vi "Transfer_Curve_2_2400.vi"(0 "File Path":path=path "C:/DATA/raj/transferdump.txt.txt", 1 "V_G Start":dbl=-0.7 format="%#.3g", 3 "V_G Finish":dbl=0.4 format="%#.3g", 4 "V_G Step Size":dbl=0.05 format="%#.3g", 5 "Preread delay (ms)":dbl=10000.0 format="%.2f", 7 "Delay between \naverages (ms)":dbl=200.0 format="%#.3f", 8 "Keithley 237 GPIB address":string="17", 9 "Software Averages":i16=5, 12 "2400":refnum<visa-resource-name>="GPIB0::24::INSTR", 13 "First bias settle (ms)":dbl=60000.0 format="%#.2f", 15 "Current Compliance\nLimit (A) Ke2400":dbl=0.1 format="%#.3e", 18 "Dimensions":T1(ring), 24 "Voltage Compliance Limit 237 (V)":dbl=10.0 format="%#.3f", 25 "Current Compliance\nLimit 237 (A)":dbl=0.1 format="%#.3f", 27 "V_DS":dbl=-0.6 format="%#_13g") -> ()   [LabVIEW 2018]
uses:
  <vilib>/Utility/file.llb/Write Delimited Spreadsheet (string).vi
  Instance           1 16Saved   JV curve .vi
  <instrlib>/Keithley 24XX/Public/Data/Read (Single Point).vi
  <vilib>/Analysis/NI_AALBase.lvlib
  <instrlib>/Keithley 24XX/Keithley 24XX.lvlib
panel:
  in  "2401":refnum<visa-resource-name>="GPIB0::22::INSTR"
  in  "Quick Burn In?":bool
  out "timer":dbl format="%#_6f"
  out "Keithley 2400":cluster{dbl[], dbl[]}(graph)={[-2.0, -1.9, -1.8, -1.7, -1.6, -1.5], [-6.6965744e-11, -6.7804984e-11, -6.685451799999999e-11, -6.6450076e-11, -6.5125542e-11, -6.7339852e-11]}
  out "I_G (A)":dbl=-6.642986e-11 format="%.2e"
  in  "Autozero?":u16(ring) items=["On", "Off", "Once"]
  in  "Measurement Speed (1 PLC)":dbl=1.0 format="%.2g"
  in  "Manual Range (Max I)":dbl=1.0
  in  "Enable Meas Auto Range":bool=TRUE
  in  "Source Mode":u16(ring) items=["Voltage", "Current"]
  in  "Return Sweep?":bool=TRUE
  out "I_DS":dbl=-1.38e-12 format="%.2e"
  out "Outputfile":path=path "C:/DATA/Mark Ziffer/test10"
  in  "Abort Scan":bool=TRUE
  out "V_G":dbl=-1.5 format="%#.2f"
  out "Keithley 237":cluster{dbl[], dbl[]}(graph)={[-2.0, -1.9, -1.8, -1.7, -1.6, -1.5], [-6.720000000000001e-13, -2.18e-13, -2.7599999999999993e-13, -8.999999999999998e-14, -1.3999999999999998e-13, -1.3800000000000002e-13]}
  # "Transfer Curve\nbased on  EL_photocurrent_JV.vi for controlling 2 Ketthleys\n\n9/2017 MZ"
  # "Software Settings"
  # "Ke237 Settings"
  # "Ke2400 Settings"
  # "Notes for IV Scan\n\n2010.07.06 - add absolute value plotter to look at log-scale current\n2010.01.07 - Modified file headers for distinguihing when imported to Igor Pro - the prefix of each header will be the file name.\n2009.01.15 - I updated the code to run on the VISA driver convention. I also modified the file saving and the option to set the\n                      graph display.\n2008.12.01 - I fixed an issue with calculations of J. It was mis-wired to divide current by wavelength, rather than active area.  BM\n\n=========================\nI added the functionality to calculate the fill factor, rectification ratio, short circuit current density, and open circuit voltage. \nAdditionally, current density (mA/cm^2) is reported in the plot window and column B of the data file, and the current (A) has been \nmoved to column C. Open circuit voltage is linearly interpolated. The max power point (mpp) for calculating fill factor is taken as \nthe data point with the highest I-V product, so this makes it only as accurate as your voltage step size, but should be fine for a decent \ndevice on the 50 mV default step size.\n\nIf you know how to use the previous versions of IV scan, \nmake sure you set these parameters before you scan:\n1) Recftification Ratio Bias - this is the +/- bias value you wish to record a rectification ratio at.\n2) Effective Area - this is the area in cm^2 of the diode mask (photoactive area) when measuring under illumination or the measured \n     area of the electrode overlap when measured in dark (regular active area).\n3) Do you want to record a separate data file for the calculated characteristics? If so, make sure the switch is on.\n\nAs of today, I couldn't figure out how to append the computed characteristics to the I-V file without experiencing formating issues, so\nI opted to just create a separate file if you want to save that info. Feel free to fix this if you know how. Check tab 3 > tab 2 > tab 9 in the\nblock diagram.\n\n2008-04-15\nB MacLeod"
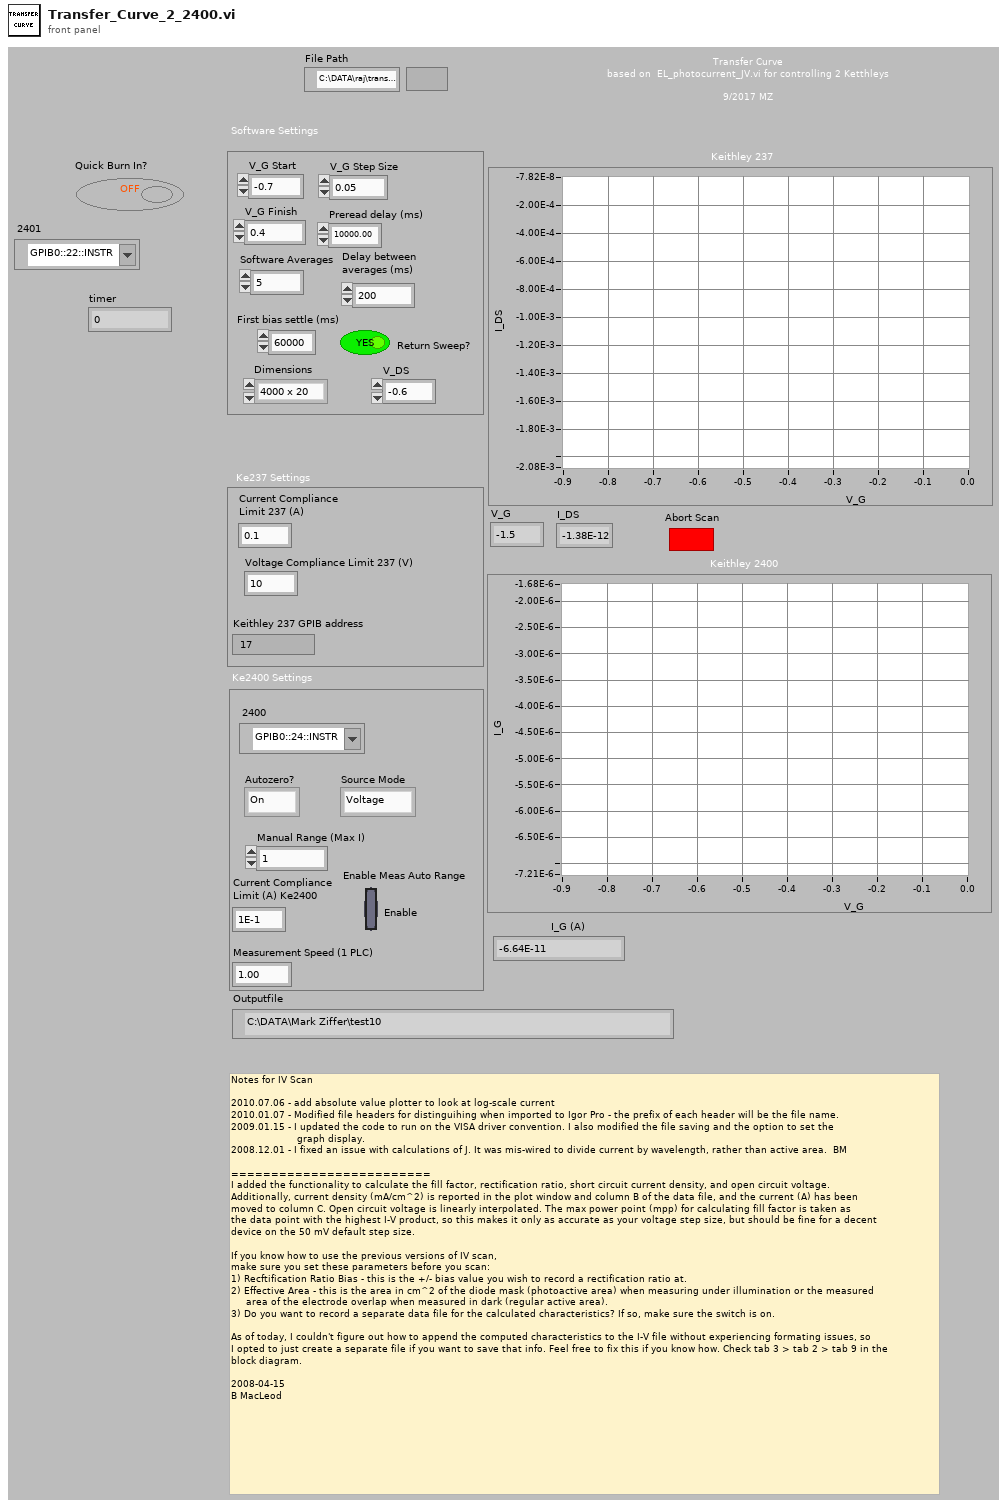
[diagram p1: front panel]
types:
  T1 = enum16{"4000 x 20", "2000 x 20", "1000 x 20", "800 x 20", "400 x 20", "200 x 20", "100 x 20"}
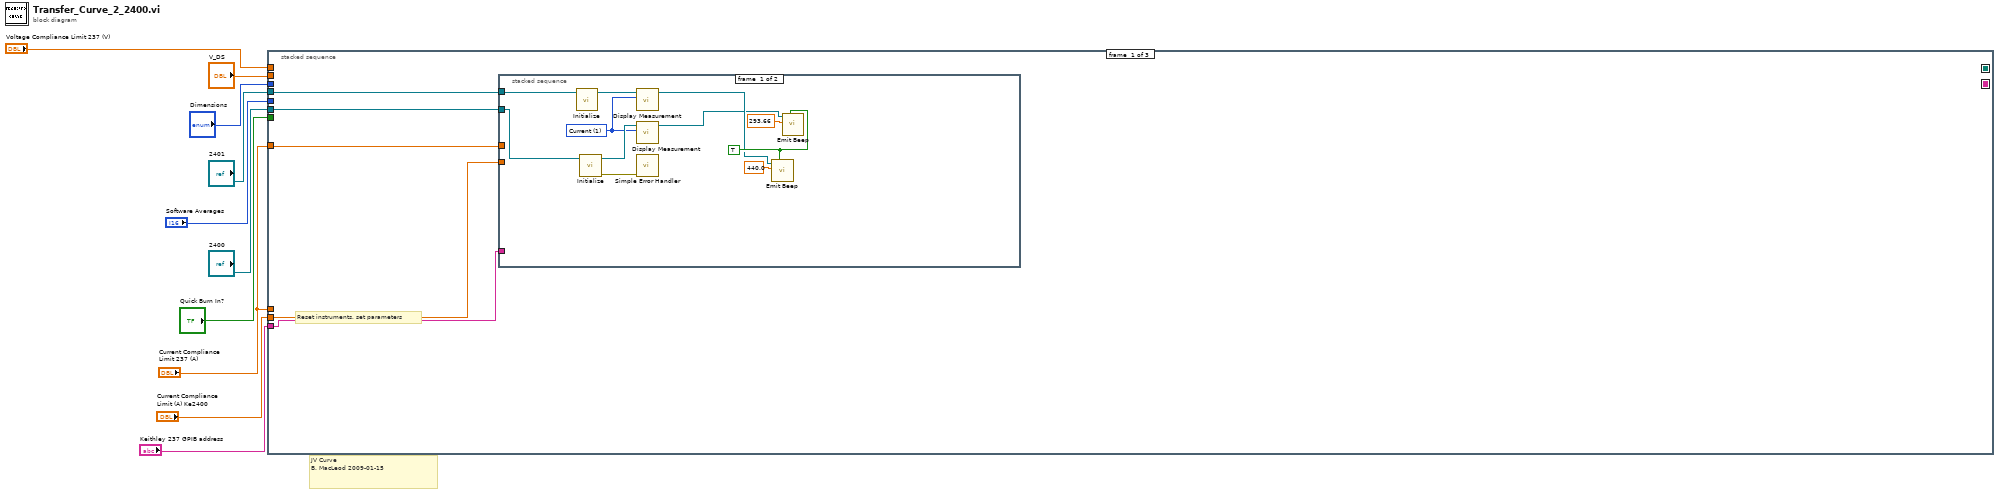
[diagram p0: block diagram]
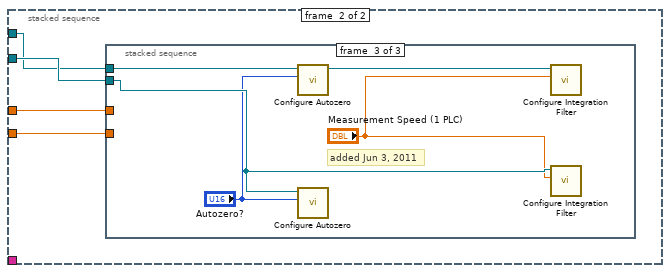
[diagram p2: hidden frame]
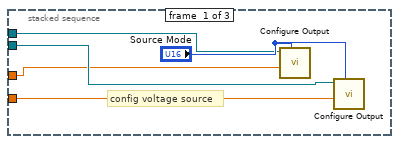
[diagram p3: hidden frame]
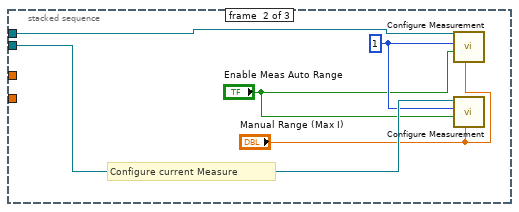
[diagram p4: hidden frame]
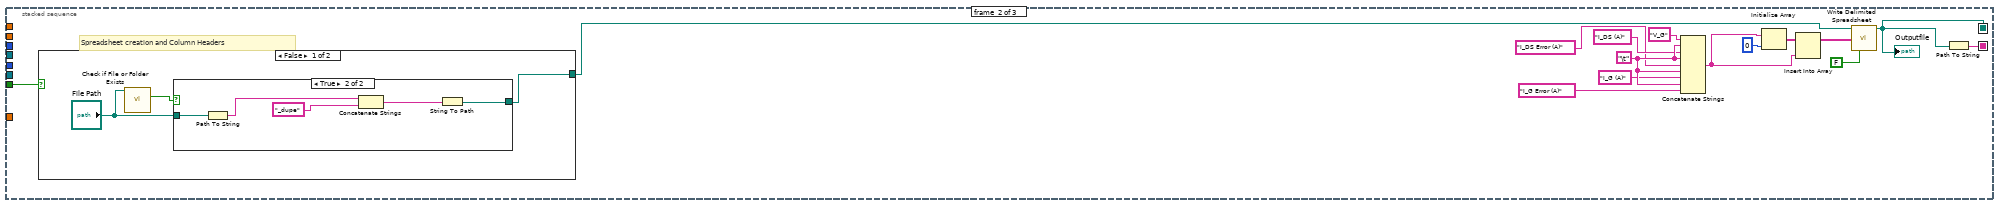
[diagram p5: hidden frame]
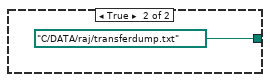
[diagram p7: hidden frame]
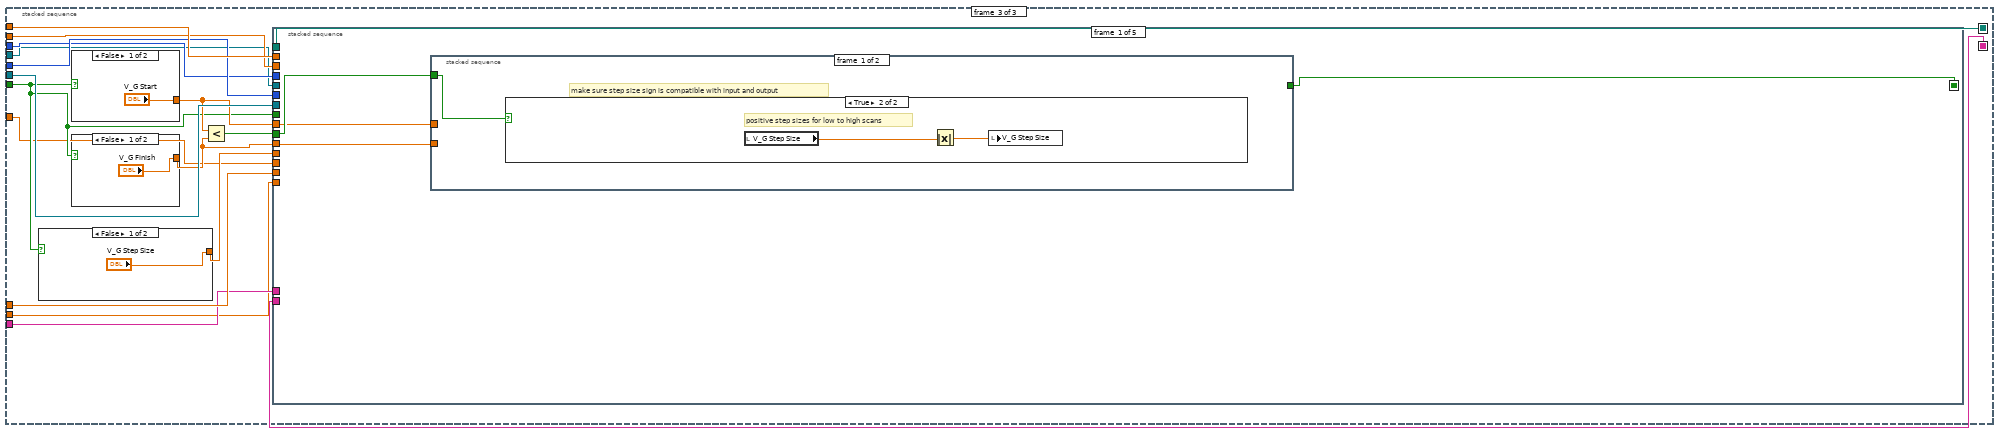
[diagram p8: hidden frame]
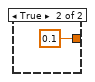
[diagram p9: hidden frame]
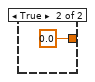
[diagram p10: hidden frame]
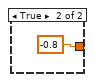
[diagram p11: hidden frame]
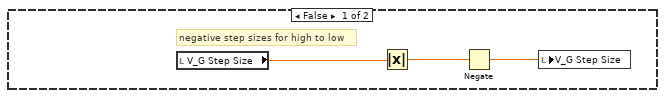
[diagram p12: hidden frame]
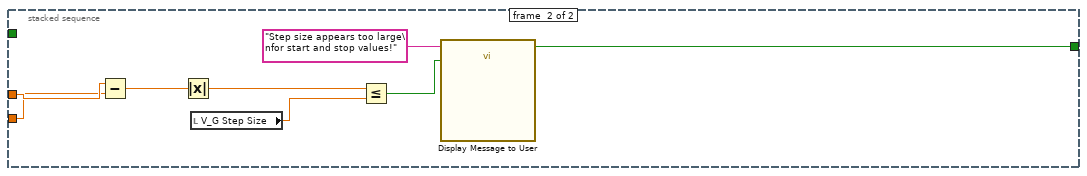
[diagram p13: hidden frame]
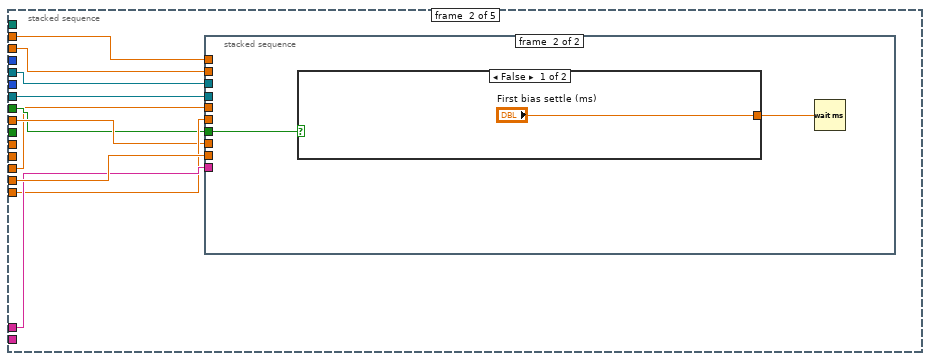
[diagram p14: hidden frame]
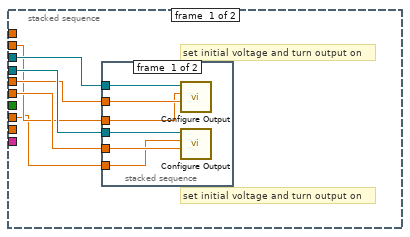
[diagram p15: hidden frame]
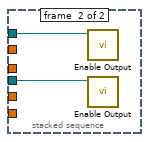
[diagram p16: hidden frame]
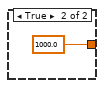
[diagram p17: hidden frame]
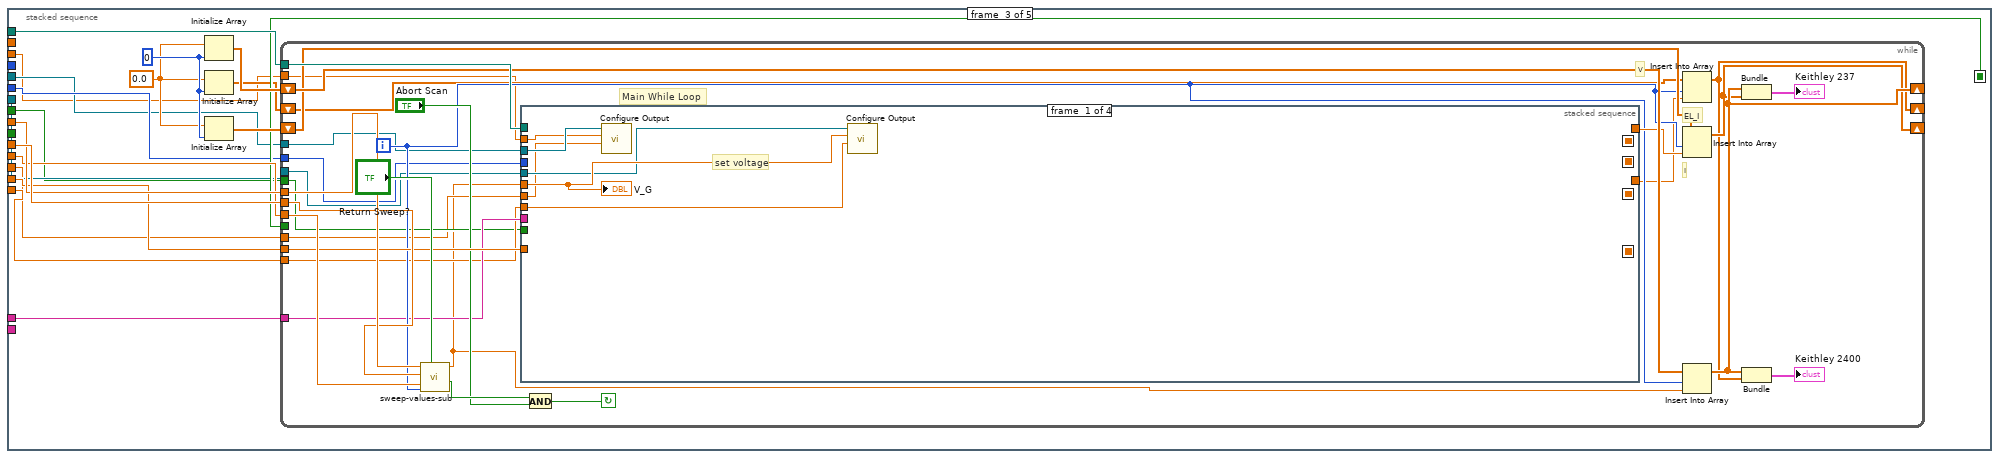
[diagram p18: hidden frame]
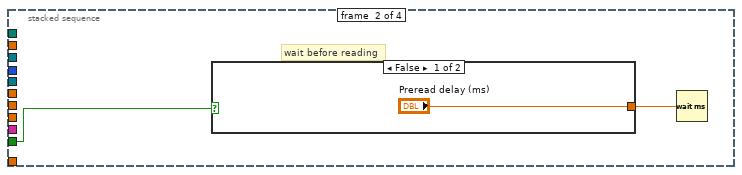
[diagram p19: hidden frame]
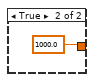
[diagram p20: hidden frame]
diagram:
  # "JV Curve\nB. MacLeod 2009-01-15"
  n1 = stacked-sequence {
    seq-local: [_ w53 _] -> [_ _ w86]
    seq-local: [_ w60 _] -> [_ _ w85]
    tunnel: "Current Compliance\nLimit 237 (A)" -> [_ _ w84]
    tunnel: "Voltage Compliance Limit 237 (V)" -> [_ _ w80]
    tunnel: "Keithley 237 GPIB address" -> [w15 _ w83]
    tunnel: "2400" -> [w12 _ w82]
    tunnel: "Current Compliance\nLimit (A) Ke2400" -> [w14 _ w81]
    tunnel: "V_DS" -> [_ _ w79]
    tunnel: "Software Averages" -> [_ _ w78]
    tunnel: "Dimensions" -> [_ _ w77]
    tunnel: "Quick Burn In?" -> [_ w46 w73]
    tunnel: "2401" -> [w11 _ w72]
    tunnel: "Current Compliance\nLimit 237 (A)" -> [w13 _ w71]
    frame #0 {
      # "Reset instruments, set parameters"
      n2 = stacked-sequence {
        tunnel: w15 -> [_ _]
        tunnel: w12 -> [w26 w30]
        tunnel: w14 -> [_ w29]
        tunnel: w11 -> [w21 w28]
        tunnel: w13 -> [_ w27]
        frame #0 {
          w20 = TRUE
          w23 = u16 1 items=["Voltage", "Current", "Resistance"] ("Displayed Measurement (0: Voltage)")
          n3 = call <instrlib>:"Initialize.vi"("VISA resource name"=w21) -> ("VISA resource name out"=w22:refnum<visa-resource-name>)  [unwired: 9 in, 1 out]
          n4 = call <instrlib>:"Initialize.vi"("VISA resource name"=w26) -> ("error out"=w24:errorcluster, "VISA resource name out"=w25:refnum<visa-resource-name>)  [unwired: 9 in]
          n5 = call <instrlib>:"Display Measurement.vi"("Displayed Measurement (0: Voltage)"=w23, "VISA resource name"=w22) -> ("VISA resource name out"=w17:refnum<visa-resource-name>)  [unwired: 8 in, 1 out]
          n6 = call <instrlib>:"Display Measurement.vi"("Displayed Measurement (0: Voltage)"=w23, "VISA resource name"=w25) -> ("VISA resource name out"=w16:refnum<visa-resource-name>)  [unwired: 8 in, 1 out]
          n7 = call <vilib>:"Simple Error Handler.vi"("error in (no error)"=w24) -> ()  [unwired: 1 in, 8 out]
          n8 = call <instrlib>:"Emit Beep.vi"("Enable Beep (F)"=w20, "Beep Frequency (300)"=440.0, "VISA resource name"=w17) -> ()  [unwired: 7 in, 2 out]
          n9 = call <instrlib>:"Emit Beep.vi"("Enable Beep (F)"=w20, "Beep Frequency (300)"=293.66, "VISA resource name"=w16) -> ()  [unwired: 7 in, 2 out]
        }
        frame #1 {
          n10 = stacked-sequence {
            tunnel: w30 -> [w35 w40 w45]
            tunnel: w29 -> [w34 _ _]
            tunnel: w28 -> [w32 w39 w44]
            tunnel: w27 -> [w31 _ _]
            frame #0 {
              # "config voltage source"
              n11 = call <instrlib>:"Configure Output.vi"("Source Mode  (0: Voltage)"="Source Mode", "Compliance  Level (0.1)"=w31, "VISA resource name"=w32) -> ()  [unwired: 3 in, 6 out]
              n12 = call <instrlib>:"Configure Output.vi"("Source Mode  (0: Voltage)"="Source Mode", "Compliance  Level (0.1)"=w34, "VISA resource name"=w35) -> ()  [unwired: 3 in, 6 out]
            }
            frame #1 {
              w37 = 1
              # "Configure current Measure"
              n13 = call <instrlib>:"Configure Measurement.vi"("Manual Range (1.0)"="Manual Range (Max I)", "Enable Auto Range (T:Enable)"="Enable Meas Auto Range", "Function (0: Volts)"=w37, "VISA resource name"=w39) -> ()  [unwired: 1 in, 7 out]
              n14 = call <instrlib>:"Configure Measurement.vi"("Manual Range (1.0)"="Manual Range (Max I)", "Enable Auto Range (T:Enable)"="Enable Meas Auto Range", "Function (0: Volts)"=w37, "VISA resource name"=w40) -> ()  [unwired: 1 in, 7 out]
            }
            frame #2 {
              # "added Jun 3, 2011"
              n15 = call <instrlib>:"Configure Autozero.vi"("Autozero  (0: On)"="Autozero?", "VISA resource name"=w44) -> ("VISA resource name out"=w43:refnum<visa-resource-name>)  [unwired: 1 in, 8 out]
              n16 = call <instrlib>:"Configure Autozero.vi"("Autozero  (0: On)"="Autozero?", "VISA resource name"=w45) -> ()  [unwired: 1 in, 9 out]
              n17 = call <instrlib>:"Configure Integration Filter.vi"("Measurement Speed (1 PLC)"="Measurement Speed (1 PLC)", "VISA resource name"=w43) -> ()  [unwired: 8 in, 2 out]
              n18 = call <instrlib>:"Configure Integration Filter.vi"("Measurement Speed (1 PLC)"="Measurement Speed (1 PLC)", "VISA resource name"=w45) -> ()  [unwired: 8 in, 2 out]
            }
          }
        }
      }
    }
    frame #1 {
      w56 = "\t"
      # "Spreadsheet creation and Column Headers"
      n19 = case shown="False" w46 {
        tunnel: [w61 path "C:/DATA/raj/transferdump.txt"] -> w47
        frame False {
          n20 = call <vilib>:"Check if File or Folder Exists.vi"("path"="File Path") -> ("file or folder exists?"=w63:bool)  [unwired: 8 in, 2 out]
          n21 = case shown="True" w63 {
            tunnel: "File Path" -> [w64 w68]
            tunnel: [w64 w65] -> w61
            frame False {
            }
            frame True {
              n22 = Path To String(path=w68) -> (string=w69:string)
              n23 = Concatenate Strings(w69, "_dupe") -> (w66:string)
              n24 = String To Path(string=w66) -> (path=w65:path)
            }
          }
        }
        frame True {
        }
      }
      n25 = Concatenate Strings("V_G", w56, "I_DS (A)", w56, "I_DS Error (A)", w56, "I_G (A)", w56, "I_G Error (A)" ("string")) -> (w58:string)
      n26 = Initialize Array(w58, 0 ("dimension size")) -> (w57:string[])
      n27 = Insert Into Array(array=w57, new element=w58) -> (w54:string[])  [unwired: 1 in]
      n28 = call-poly <vilib>:"Write Delimited Spreadsheet.vi"("file path (dialog if empty)"=w47, "1D data"=w54, "transpose? (no:F)"=FALSE ("append to file? (new file:F)")) -> ("new file path (Not A Path if cancelled)"=w53:path)  [unwired: 11 in, 1 out]
      "Outputfile" <- w53
      n29 = Path To String(path=w53) -> (string=w60:string)
    }
    frame #2 {
      n30 = case shown="False" w73 {
        tunnel: ["V_G Step Size" 0.1] -> w74
        frame False {
        }
        frame True {
        }
      }
      n31 = case shown="False" w73 {
        tunnel: ["V_G Start" -0.8] -> w76
        frame False {
        }
        frame True {
        }
      }
      n32 = case shown="False" w73 {
        tunnel: ["V_G Finish" 0.0] -> w75
        frame False {
        }
        frame True {
        }
      }
      n33 = Less?(x=w76, y=w75) -> (x < y?=w87:bool)
      n34 = stacked-sequence {
        seq-local: [w94 _ _ _ _] -> [_ _ w151 _ _]
        tunnel: w87 -> [w97 _ _ _ _]
        tunnel: w76 -> [w96 w116 w157 _ _]
        tunnel: w75 -> [w95 _ w158 _ _]
        tunnel: w74 -> [_ _ w156 _ _]
        tunnel: w86 -> [_ _ w155 w239 _]
        tunnel: w85 -> [_ _ _ _ _]
        tunnel: w84 -> [_ w121 w152 _ _]
        tunnel: w83 -> [_ w120 w150 _ w295]
        tunnel: w82 -> [_ w118 w149 _ w294]
        tunnel: w81 -> [_ w119 w145 _ _]
        tunnel: w80 -> [_ w117 _ _ _]
        tunnel: w79 -> [_ w115 w141 w240 _]
        tunnel: w78 -> [_ _ w144 w238 _]
        tunnel: w77 -> [_ _ _ w237 _]
        tunnel: w73 -> [_ w114 w143 _ _]
        tunnel: w72 -> [_ w113 w142 _ _]
        tunnel: w71 -> [_ w112 w140 _ _]
        frame #0 {
          n35 = stacked-sequence {
            tunnel: w97 -> [w98 _]
            tunnel: w96 -> [_ w111]
            tunnel: w95 -> [_ w110]
            tunnel: [_ w104] -> w94
            frame #0 {
              # "make sure step size sign is compatible with input and output"
              n36 = case shown="True" w98 {
                frame False {
                  # "negative step sizes for high to low"
                  n37 = local read "V_G Step Size"() -> (w101:dbl)
                  n38 = Absolute Value(x=w101) -> (abs(x)=w100:dbl)
                  n39 = Negate(x=w100) -> (-x=w99:dbl)
                  n40 = local write "V_G Step Size"(w99) -> ()
                }
                frame True {
                  # "positive step sizes for low to high scans"
                  n41 = local read "V_G Step Size"() -> (w103:dbl)
                  n42 = Absolute Value(x=w103) -> (abs(x)=w102:dbl)
                  n43 = local write "V_G Step Size"(w102) -> ()
                }
              }
            }
            frame #1 {
              n44 = Subtract(x=w111, y=w110) -> (x-y=w109:dbl)
              n45 = Absolute Value(x=w109) -> (abs(x)=w108:dbl)
              n46 = local read "V_G Step Size"() -> (w107:dbl)
              n47 = Less Or Equal?(x=w108, y=w107) -> (x <= y?=w105:bool)
              n48 = call "Display Message to User"("Enable"=w105, "Message"="Step size appears too large\nfor start and stop values!") -> ("OK"=w104:bool)  [unwired: 1 in, 8 out]
            }
          }
        }
        frame #1 {
          n49 = stacked-sequence {
            tunnel: w121 -> [_ _]
            tunnel: w120 -> [_ _]
            tunnel: w119 -> [w127 _]
            tunnel: w118 -> [w126 _]
            tunnel: w117 -> [_ _]
            tunnel: w116 -> [w122 _]
            tunnel: w115 -> [w123 _]
            tunnel: w114 -> [_ w137]
            tunnel: w113 -> [w125 _]
            tunnel: w112 -> [w124 _]
            frame #0 {
              # "set initial voltage and turn output on"
              # "set initial voltage and turn output on"
              n50 = stacked-sequence {
                tunnel: w127 -> [w133 _]
                tunnel: w126 -> [w132 w135]
                tunnel: w125 -> [w131 w134]
                tunnel: w124 -> [w130 _]
                tunnel: w123 -> [w129 _]
                tunnel: w122 -> [w128 _]
                frame #0 {
                  n51 = call <instrlib>:"Configure Output.vi"("Compliance  Level (0.1)"=w130, "Output Level (0)"=w129, "VISA resource name"=w131) -> ()  [unwired: 3 in, 6 out]
                  n52 = call <instrlib>:"Configure Output.vi"("Compliance  Level (0.1)"=w133, "Output Level (0)"=w128, "VISA resource name"=w132) -> ()  [unwired: 3 in, 6 out]
                }
                frame #1 {
                  n53 = call <instrlib>:"Enable Output.vi"("VISA resource name"=w134) -> ()  [unwired: 2 in, 9 out]
                  n54 = call <instrlib>:"Enable Output.vi"("VISA resource name"=w135) -> ()  [unwired: 2 in, 9 out]
                }
              }
            }
            frame #1 {
              n55 = case shown="False" w137 {
                tunnel: ["First bias settle (ms)" 1000.0] -> w136
                frame False {
                }
                frame True {
                }
              }
              n56 = Wait (ms)(milliseconds to wait=w136) -> ()  [unwired: 1 out]
            }
          }
        }
        frame #2 {
          w148 = 0
          w147 = 0.0
          n57 = Initialize Array(w147, w148) -> (w154:dbl[])
          n58 = Initialize Array(w147, w148) -> (w146:dbl[])
          n59 = Initialize Array(w147, w148) -> (w153:dbl[])
          n60 = while {
            shift-left: w153 -> [w184]
            shift-right: [w172] -> _
            shift-left: w154 -> [w185]
            shift-right: [w175] -> _
            tunnel: w155 -> [w186]
            tunnel: w156 -> [w183]
            tunnel: w157 -> [w182]
            tunnel: w158 -> [w181]
            tunnel: w152 -> [w179]
            tunnel: w151 -> [_]
            shift-right: [w171] -> _
            shift-left: w146 -> [w167]
            tunnel: w150 -> [w170]
            tunnel: w149 -> [w169]
            tunnel: w145 -> [w165]
            tunnel: w144 -> [w164]
            tunnel: w143 -> [w163]
            tunnel: w142 -> [w162]
            tunnel: w141 -> [w161]
            tunnel: w140 -> [w160]
            i -> [w173]
            stop <- w177 continue-if-true
            # "EL_I"
            # "Main While Loop"
            # "V"
            # "I"
            n61 = call "sweep-values-sub.vi"("Forward/Reverse"="Return Sweep?", "Point Number"=w173, "Step Size"=w183, "Sweep Stop"=w181, "Sweep Start"=w182) -> ("Active"=w178:bool, "Output"=w159:dbl)  [unwired: 2 out]
            n62 = stacked-sequence {
              seq-local: [_ _ w207 _] -> [_ _ _ w221]
              seq-local: [_ _ w202 _] -> [_ _ _ w222]
              seq-local: [_ _ w204 _] -> [_ _ _ w220]
              seq-local: [_ _ w203 _] -> [_ _ _ w219]
              tunnel: [_ _ w202 _] -> w174
              tunnel: w159 -> [w193 _ _ w233]
              tunnel: w186 -> [_ _ _ w224]
              tunnel: w179 -> [_ _ _ _]
              tunnel: w170 -> [_ _ w206 _]
              tunnel: w169 -> [w191 _ w205 _]
              tunnel: [_ _ w204 _] -> w168
              tunnel: w165 -> [w192 _ _ _]
              tunnel: w164 -> [_ _ w201 _]
              tunnel: w163 -> [_ w194 _ _]
              tunnel: w162 -> [w190 _ w199 _]
              tunnel: w161 -> [w189 _ _ _]
              tunnel: w160 -> [w188 _ _ _]
              frame #0 {
                # "set voltage"
                n63 = call <instrlib>:"Configure Output.vi"("Compliance  Level (0.1)"=w188, "Output Level (0)"=w189, "VISA resource name"=w190) -> ()  [unwired: 3 in, 6 out]
                n64 = call <instrlib>:"Configure Output.vi"("Compliance  Level (0.1)"=w192, "Output Level (0)"=w193, "VISA resource name"=w191) -> ()  [unwired: 3 in, 6 out]
                "V_G" <- w193
              }
              frame #1 {
                # "wait before reading"
                n65 = case shown="False" w194 {
                  tunnel: ["Preread delay (ms)" 1000.0] -> w195
                  frame False {
                  }
                  frame True {
                  }
                }
                n66 = Wait (ms)(milliseconds to wait=w195) -> ()  [unwired: 1 out]
              }
              frame #2 {
                # "I_DS"
                # "I_G"
                # "read values"
                n67 = for {
                  N: w201 -> [_]
                  tunnel: w206 -> [w212]
                  tunnel: w205 -> [w211]
                  tunnel: [w210] -> w200 mode=indexing
                  tunnel: w199 -> [w209]
                  tunnel: [w208] -> w198 mode=indexing
                  n68 = stacked-sequence {
                    tunnel: w212 -> [_ _]
                    tunnel: w211 -> [w216 _]
                    tunnel: [w215 _] -> w210
                    tunnel: w209 -> [w214 _]
                    tunnel: [w213 _] -> w208
                    frame #0 {
                      n69 = call-poly <instrlib>:"Read.vi"("VISA resource name"=w214) -> ("Current"=w213:sgl)  [unwired: 8 in, 6 out]
                      "I_DS" <- w213
                      n70 = call-poly <instrlib>:"Read.vi"("VISA resource name"=w216) -> ("Current"=w215:sgl)  [unwired: 8 in, 6 out]
                      "I_G (A)" <- w215
                    }
                    frame #1 {
                      n71 = Wait (ms)(milliseconds to wait="Delay between \naverages (ms)") -> (millisecond timer value=→"timer":u32)
                    }
                  }
                }
                n72 = call <vilib>:"Std Deviation and Variance.vi"("X"=w200) -> ("mean"=w204:dbl, "standard deviation"=w203:dbl)  [unwired: 1 in, 1 out]
                n73 = call <vilib>:"Std Deviation and Variance.vi"("X"=w198) -> ("mean"=w202:dbl, "standard deviation"=w207:dbl)  [unwired: 1 in, 1 out]
              }
              frame #3 {
                w228 = "\t"
                # "I_G"
                # "write data to file"
                # "X"
                n74 = Format Into String(format string="%#f", w233) -> (resulting string=w231:string)  [unwired: 2 in, 1 out]
                n75 = Number To Exponential String(number=w222) -> (E-format string=w234:string)  [unwired: 3 out]
                n76 = Number To Exponential String(number=w221) -> (E-format string=w230:string)  [unwired: 3 out]
                n77 = Number To Exponential String(number=w219) -> (E-format string=w226:string)  [unwired: 3 out]
                n78 = Number To Exponential String(number=w220) -> (E-format string=w227:string)  [unwired: 3 out]
                n79 = Concatenate Strings(w231, w228, w234, w228, w230, w228, w227, w228, w226) -> (w229:string)
                n80 = Build Array(w229) -> (w225:string[])
                n81 = call-poly <vilib>:"Write Delimited Spreadsheet.vi"("file path (dialog if empty)"=w224, "1D data"=w225, "append to file? (new file:F)"=TRUE) -> ()  [unwired: 11 in, 2 out]
              }
            }
            n82 = Compound Arithmetic op=AND(w178, "Abort Scan") -> (w177:bool)
            n83 = Insert Into Array(array=w167, index=w173, new element=w168) -> (w171:dbl[])
            n84 = Insert Into Array(array=w184, index=w173, new element=w174) -> (w172:dbl[])
            n85 = Insert Into Array(array=w185, index=w173, new element=w159) -> (w175:dbl[])
            n86 = Bundle(w175, w172) -> (→"Keithley 237":cluster{dbl[], dbl[]})  [unwired: 1 out]
            n87 = Bundle(w175, w171) -> (→"Keithley 2400":cluster{dbl[], dbl[]})  [unwired: 1 out]
          }
        }
        frame #3 {
          n88 = case shown="\"2000 x 20\"" w237 {
            tunnel: [4000 2000 1000 800 400 200 100] -> w236
            tunnel: [20 20 20 20 20 20 20] -> w235
            frame "4000 x 20", Default {
            }
            frame "2000 x 20" {
            }
            frame "1000 x 20" {
            }
            frame "800 x 20" {
            }
            frame "400 x 20" {
            }
            frame "200 x 20" {
            }
            frame "100 x 20" {
            }
          }
          n89 = stacked-sequence {
            tunnel: w240 -> [_ w266 _ _ _]
            tunnel: w239 -> [w255 w264 w270 w285 w287]
            tunnel: w238 -> [_ _ w272 _ _]
            tunnel: w236 -> [_ _ _ w280 _]
            tunnel: w235 -> [_ _ _ _ w286]
            frame #0 {
              w260 = ""
              w259 = "\t"
              n90 = Concatenate Strings(w260, w259, w260, w259) -> (w256:string)
              n91 = Build Array(w256) -> (w258:string[])
              n92 = call-poly <vilib>:"Write Delimited Spreadsheet.vi"("file path (dialog if empty)"=w255, "1D data"=w258, "append to file? (new file:F)"=TRUE) -> ()  [unwired: 11 in, 2 out]
            }
            frame #1 {
              w267 = "\t"
              n93 = Number To Fractional String(number=w266, precision (6)=3) -> (F-format string=w265:string)  [unwired: 2 in]
              n94 = Concatenate Strings("V_DS = ", w267, w265, w267) -> (w268:string)
              n95 = Build Array(w268) -> (w263:string[])
              n96 = call-poly <vilib>:"Write Delimited Spreadsheet.vi"("file path (dialog if empty)"=w264, "1D data"=w263, "append to file? (new file:F)"=TRUE) -> ()  [unwired: 11 in, 2 out]
            }
            frame #2 {
              w275 = "\t"
              n97 = Number To Decimal String(number=w272) -> (decimal integer string=w271:string)  [unwired: 1 in]
              n98 = Concatenate Strings("Number of Averages = ", w275, w271, w275) -> (w276:string)
              n99 = Build Array(w276) -> (w274:string[])
              n100 = call-poly <vilib>:"Write Delimited Spreadsheet.vi"("file path (dialog if empty)"=w270, "1D data"=w274, "append to file? (new file:F)"=TRUE) -> ()  [unwired: 11 in, 2 out]
            }
            frame #3 {
              w282 = "\t"
              n101 = Number To Decimal String(number=w280) -> (decimal integer string=w281:string)  [unwired: 1 in]
              n102 = Concatenate Strings("Width/um =", w282, w281, w282) -> (w279:string)
              n103 = Build Array(w279) -> (w278:string[])
              n104 = call-poly <vilib>:"Write Delimited Spreadsheet.vi"("file path (dialog if empty)"=w285, "1D data"=w278, "append to file? (new file:F)"=TRUE) -> ()  [unwired: 11 in, 2 out]
            }
            frame #4 {
              w288 = "\t"
              n105 = Number To Decimal String(number=w286) -> (decimal integer string=w291:string)  [unwired: 1 in]
              n106 = Concatenate Strings("Length/um =", w288, w291, w288) -> (w292:string)
              n107 = Build Array(w292) -> (w293:string[])
              n108 = call-poly <vilib>:"Write Delimited Spreadsheet.vi"("file path (dialog if empty)"=w287, "1D data"=w293, "append to file? (new file:F)"=TRUE) -> ()  [unwired: 11 in, 2 out]
            }
          }
        }
        frame #4 {
          # "reset instrument at end of sweep"
          n109 = call <instrlib>:"Reset.vi"("VISA resource name"=w294) -> ()  [unwired: 9 in, 2 out]
          n110 = call <userlib>:"Keith 237 Reset.vi"("GPIB address"=w295) -> ()  [unwired: 1 in, 1 out]
        }
      }
    }
  }
